vi "File_Build Graphic Cluster from File Data.vi"(8 "Error":errorcluster, 11 "File Data":T1) -> (0 "Error Out":errorcluster, 3 "Path And Icon Out":T2)   [LabVIEW 2021]
uses:
  TypeDefs/Cluster_Path&Icon.ctl
  TypeDefs/Cluster_IconFilename.ctl
  vi.lib/LabVIEW Icon API/lv_icon/lv_icon.lvlib
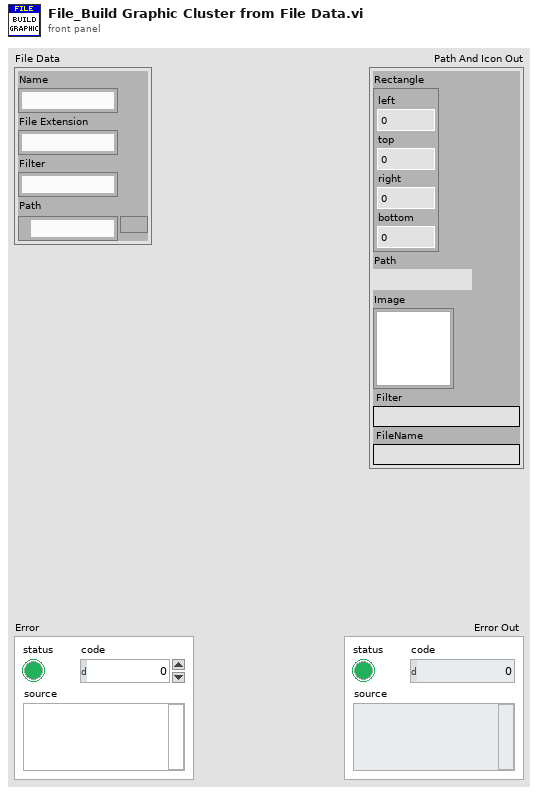
[diagram p1: front panel]
types:
  T1 = typedef "Cluster_IconFilename.ctl" = cluster{"Name":string, "File Extension  ":string, "Filter":string, "Path":path}
  T2 = typedef "Cluster_Path&Icon.ctl" = cluster{"Rectangle":cluster{"left":i16, "top":i16, "right":i16, "bottom":i16}, "Path":path, "Image":picture, "Filter":string, "FileName":string}
  T3 = typedef "imagedata.ctl" = cluster{"image type":i32, "image depth":i32, "image":u8[], "mask":u8[], "colors":u32[], "Rectangle":cluster{"left":i16, "top":i16, "right":i16, "bottom":i16}}
  T4 = cluster{"left":i16, "top":i16, "right":i16, "bottom":i16}
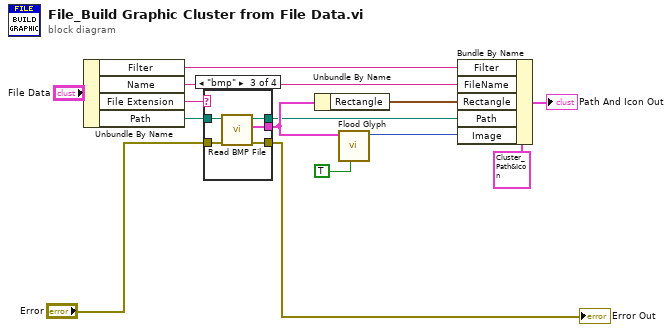
[diagram p0: block diagram]
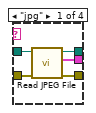
[diagram p2: hidden frame]
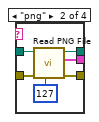
[diagram p3: hidden frame]
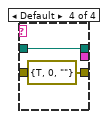
[diagram p4: hidden frame]
diagram:
  n1 = Unbundle By Name("File Data") -> ("Filter"=w10:string, "Name"=w11:string, "File Extension"=w5:string, "Path"=w3:path)
  n2 = case shown="\"bmp\"" w5 {
    tunnel: [w19 w25 w30 errorcluster {"status"=TRUE, "code"=0, "source"=""} ("error out")] -> w6
    tunnel: [w18 w24 w29 _] -> w4
    tunnel: [w16 w22 w27 w32] -> w1
    tunnel: w3 -> [w17 w23 w28 w32]
    tunnel: "Error" -> [w15 w20 w26 _]
    frame "jpg" {
      n3 = call <vilib>:"Read JPEG File.vi"("error in (no error)"=w15, "path to JPEG file"=w17) -> ("error out"=w19:errorcluster, "image data"=w18:T3, "path"=w16:path)  [unwired: 7 out]
    }
    frame "png" {
      n4 = call <vilib>:"Read PNG File.vi"("Transparency Thresh"=u8 127, "error in (no error)"=w20, "path to PNG file"=w23) -> ("error out"=w25:errorcluster, "image data"=w24:T3, "path"=w22:path)  [unwired: 6 out]
    }
    frame "bmp" {
      n5 = call <vilib>:"Read BMP File.vi"("error in (no error)"=w26, "path to BMP file"=w28) -> ("error out"=w30:errorcluster, "image data"=w29:T3, "path"=w27:path)  [unwired: 7 out]
    }
    frame Default {
    }
  }
  "Error Out" <- w6
  n6 = Unbundle By Name(w4) -> ("Rectangle"=w12:T4)
  n7 = call "Flood Glyph.vi"("Use New Fill Algorithm? (F)"=TRUE, "Image Data"=w4) -> ("Pic Out"=w13:picture)  [unwired: 9 out]
  n8 = Bundle By Name(cluster=T2 {"Rectangle"={"left"=0, "top"=0, "right"=0, "bottom"=0}, "Path"=path "", "Image"=bytes[0], "Filter"="", "FileName"=""} ("Path and Icon"), "Filter"=w10, "FileName"=w11, "Rectangle"=w12, "Path"=w1, "Image"=w13) -> (→"Path And Icon Out":T2)
